vi "SLM_display A.vi"(1 "SLM Settings":T1={"resizeTo"=enum."Width of Display", "displayOn"=enum."All 3rd Monitor", "Top Left of Hologram"={"Horizontal"=60, "Vertical"=-210}}, 2 "SLM colour coding":enum16{"8-bit", "10-bit (Santec)"}(ring)=enum."10-bit (Santec)", 4 "Hologram":dbl[][](array[numeric])=array256x256[65536 elements]) -> (0 "SLM A":picture)   [LabVIEW 2024]
uses:
  typeDefs/slmSettings.ctl
  <vilib>/picture/picture.llb/Draw 8-Bit Pixmap.vi
  <vilib>/picture/picture.llb/Draw True-Color Pixmap.vi
panel:
  in  "Blazing Function 2":u8[](array[numeric])=[1, 2, 3, 4, 5, 6, 7, 8, 9, 10, 10, 11, 12, 13, 14, 15, 16, 17, 18, 19, 20, 21, 22, 23, 24, 25, 26, 27, 28, 29, 30, 31, 32, 32, 33, 34, 35, 36, 37, 38, 39, 40, 41, 42, 43, 44, 45, 46, 47, 48, 49, 50, 51, 52, 53, 54, 55, 56, 57, 58, 59, 60, 61, 61, 62, 63, 64, 65, 66, 67, 68, 69, 70, 71, 72, 73, 74, 75, 76, 77, 78, 79, 80, 81, 83, 84, 85, 86, 87, 88, 89, 90, 91, 92, 93, 94, 95, 96, 97, 98, 99, 100, 101, 102, 103, 104, 105, 106, 107, 108, 109, 111, 112, 113, 114, 115, 116, 117, 118, 119, 120, 121, 122, 123, 124, 125, 126, 127, 128, 129, 130, 131, 133, 134, 135, 136, 137, 138, 139, 140, 141, 142, 143, 144, 145, 146, 147, 148, 149, 150, 151, 152, 153, 154, 155, 156, 157, 158, 159, 160, 161, 162, 163, 164, 165, 166, 167, 168, 169, 170, 171, 172, 173, 174, 175, 176, 177, 178, 179, 180, 181, 182, 183, 184, 185, 186, 187, 188, 189, 190, 191, 192, 193, 194, 195, 196, 197, 198, 198, 199, 200, 201, 202, 203, 204, 205, 206, 207, 208, 209, 210, 211, 212, 213, 214, 215, 216, 217, 218, 219, 219, 220, 221, 222, 223, 224, 225, 226, 227, 228, 229, 230, 231, 232, 233, 234, 235, 236, 237, 238, 238, 239, 240, 241, 242, 243, 244, 245, 246, 247, 248, 249, 250, 251, 252, 253]
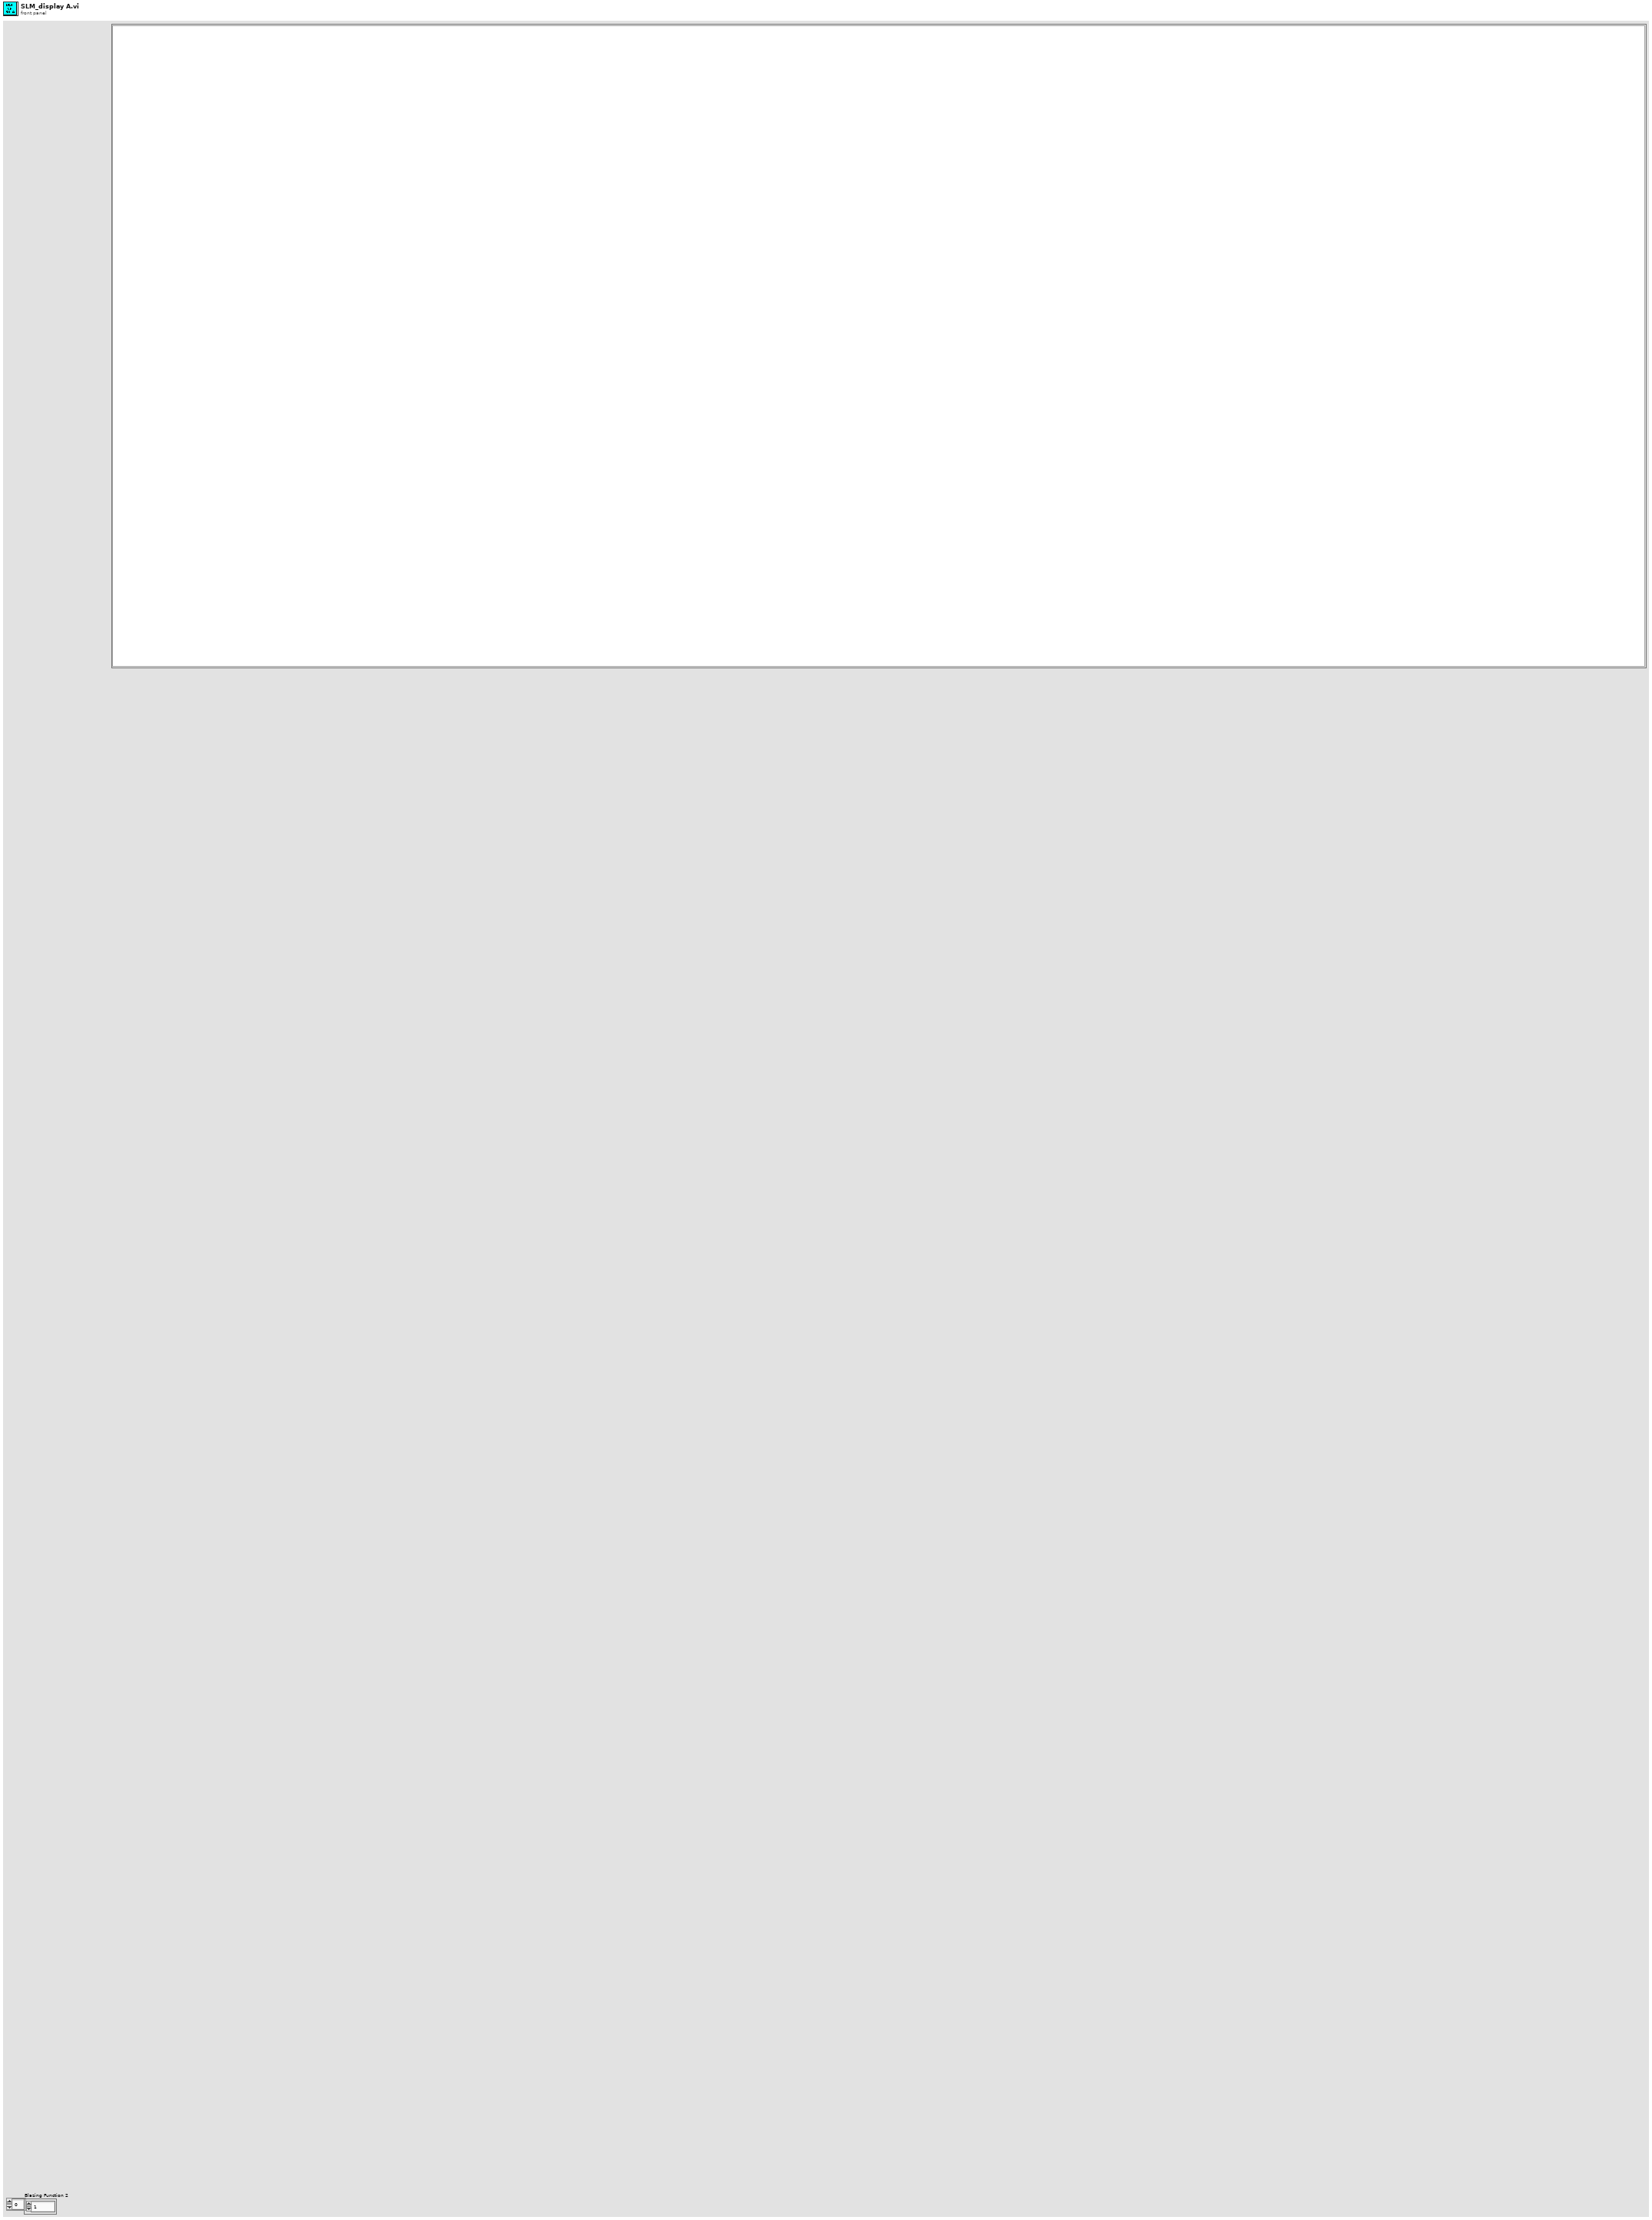
[diagram p1: front panel]
types:
  T1 = typedef "slmSettings.ctl" = cluster{"resizeTo":enum16{"No Resize", "Width of Display", "Height of Display"}, "displayOn":enum16{"Default", "All 1st Monitor", "All 2nd Monitor", "All 3rd Monitor", "All 4th Monitor"}, "Top Left of Hologram":cluster{"Horizontal":i16, "Vertical":i16}}
  T2 = enum16{"No Resize", "Width of Display", "Height of Display"}
  T3 = enum16{"Default", "All 1st Monitor", "All 2nd Monitor", "All 3rd Monitor", "All 4th Monitor"}
  T4 = typedef "LVRectTypeDef.ctl" = cluster{"Left":i16, "Top":i16, "Right":i16, "Bottom":i16}
  T5 = typedef "LVAllMonitorsDisplayTypeDef.ctl" = cluster{"Bounds":cluster{"Left":i16, "Top":i16, "Right":i16, "Bottom":i16}, "Depth":i16}[]
  T6 = cluster{"Bounds":cluster{"Left":i16, "Top":i16, "Right":i16, "Bottom":i16}, "Depth":i16}
  T7 = cluster{"Left":i16, "Top":i16, "Right":i16, "Bottom":i16}
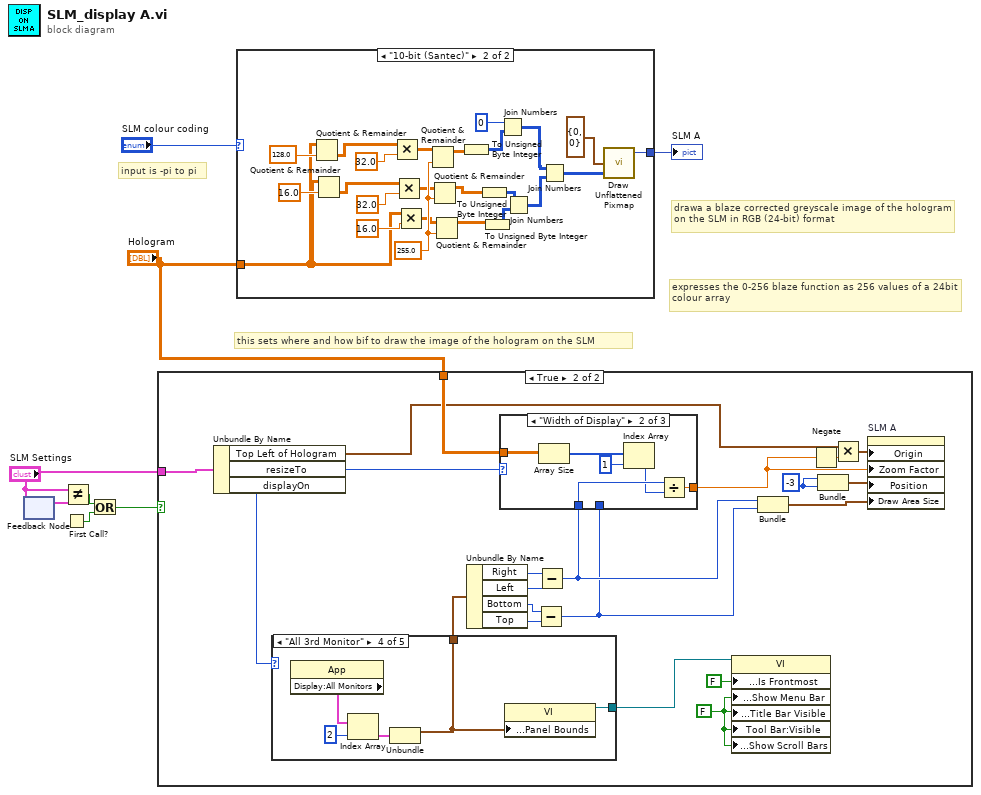
[diagram p0: block diagram]
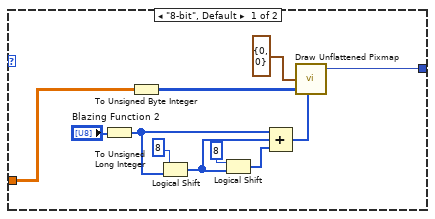
[diagram p2: hidden frame]
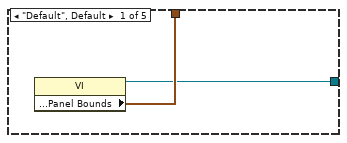
[diagram p4: hidden frame]
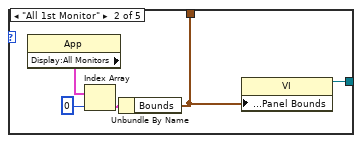
[diagram p5: hidden frame]
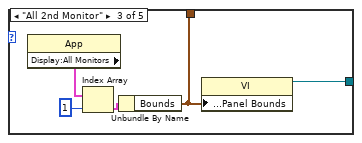
[diagram p6: hidden frame]
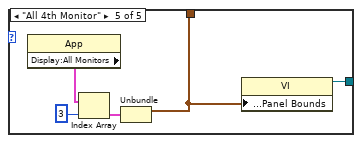
[diagram p7: hidden frame]
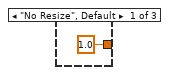
[diagram p8: hidden frame]
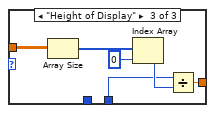
[diagram p9: hidden frame]
diagram:
  # "this sets where and how bif to draw the image of the hologram on the SLM"
  # "drawa a blaze corrected greyscale image of the hologram on the SLM in RGB (24-bit) format"
  # "input is -pi to pi"
  # "expresses the 0-256 blaze function as 256 values of a 24bit colour array"
  n1 = feedback-in #1("SLM Settings") -> ()
  n2 = feedback #1() -> (w8:T1)  [unwired: 1 in]
  n3 = First Call?() -> (First Call?: T/F=w7:bool)
  n4 = Not Equal?(x="SLM Settings", y=w8) -> (x != y?=w6:bool)
  n5 = Or(x=w6, y=w7) -> (x .or. y?=w5:bool)
  n6 = case shown="True" w5 {
    tunnel: "Hologram" -> [_ w24]
    tunnel: "SLM Settings" -> [_ w10]
    frame False {
    }
    frame True {
      w19 = i16 -3 ("x-y")
      w28 = FALSE ("Front Panel Window:Size To Screen")
      n7 = Unbundle By Name(w10) -> ("Top Left of Hologram"=w9:cluster{"Horizontal":i16, "Vertical":i16}, "resizeTo"=w26:T2, "displayOn"=w12:T3)
      n8 = case shown="\"All 3rd Monitor\"" w12 {
        tunnel: [w31 w33 w37 w43 w47] -> w27
        tunnel: [w30 w32 w38 w42 w48] -> w25
        frame "Default", Default {
          n9 = property class="VI"() -> (reference out=w30:refnum<vi>, "Front Panel Window:Panel Bounds"=w31:T4)  [unwired: 2 in, 1 out]
        }
        frame "All 1st Monitor" {
          n10 = property class="App"() -> ("Display:All Monitors"=w35:T5)  [unwired: 2 in, 2 out]
          n11 = Index Array(array=w35, index=0) -> (element=w34:T6)
          n12 = Unbundle By Name(w34) -> ("Bounds"=w33:T7)
          n13 = property class="VI"("Front Panel Window:Panel Bounds"=w33) -> (reference out=w32:refnum<vi>)  [unwired: 2 in, 1 out]
        }
        frame "All 2nd Monitor" {
          n14 = property class="App"() -> ("Display:All Monitors"=w40:T5)  [unwired: 2 in, 2 out]
          n15 = Index Array(array=w40, index=1) -> (element=w39:T6)
          n16 = Unbundle By Name(w39) -> ("Bounds"=w37:T7)
          n17 = property class="VI"("Front Panel Window:Panel Bounds"=w37) -> (reference out=w38:refnum<vi>)  [unwired: 2 in, 1 out]
        }
        frame "All 3rd Monitor" {
          n18 = property class="App"() -> ("Display:All Monitors"=w45:T5)  [unwired: 2 in, 2 out]
          n19 = Index Array(array=w45, index=2) -> (element=w44:T6)
          n20 = Unbundle(w44) -> ("Bounds"=w43:T7)  [unwired: 1 out]
          n21 = property class="VI"("Front Panel Window:Panel Bounds"=w43) -> (reference out=w42:refnum<vi>)  [unwired: 2 in, 1 out]
        }
        frame "All 4th Monitor" {
          n22 = property class="App"() -> ("Display:All Monitors"=w50:T5)  [unwired: 2 in, 2 out]
          n23 = Index Array(array=w50, index=3) -> (element=w49:T6)
          n24 = Unbundle(w49) -> ("Bounds"=w47:T7)  [unwired: 1 out]
          n25 = property class="VI"("Front Panel Window:Panel Bounds"=w47) -> (reference out=w48:refnum<vi>)  [unwired: 2 in, 1 out]
        }
      }
      n26 = Unbundle By Name(w27) -> ("Right"=w15:i16, "Left"=w14:i16, "Bottom"=w17:i16, "Top"=w16:i16)
      n27 = Subtract(x=w17, y=w16) -> (x-y=w11:i16)
      n28 = Subtract(x=w15, y=w14) -> (x-y=w13:i16)
      n29 = case shown="\"Width of Display\"" w26 {
        tunnel: w13 -> [_ w56 _]
        tunnel: [1.0 w55 w62] -> w23
        tunnel: w11 -> [_ _ w60]
        tunnel: w24 -> [_ w53 w59]
        frame "No Resize", Default {
        }
        frame "Width of Display" {
          n30 = Array Size(array=w53) -> (size(s)=w58:i32[])
          n31 = Index Array(array=w58, index=1) -> (element=w54:i32)
          n32 = Divide(x=w56, y=w54) -> (x/y=w55:dbl)
        }
        frame "Height of Display" {
          n33 = Array Size(array=w59) -> (size(s)=w64:i32[])
          n34 = Index Array(array=w64, index=0) -> (element=w61:i32)
          n35 = Divide(x=w60, y=w61) -> (x/y=w62:dbl)
        }
      }
      n36 = property class="VI"(reference=w25, "Front Panel Window:Is Frontmost"=FALSE ("Front Panel Window:Size To Screen"), "Front Panel Window:Show Menu Bar"=w28, "Front Panel Window:Title Bar Visible"=w28, "Tool Bar:Visible"=w28, "Front Panel Window:Show Scroll Bars"=w28) -> ()  [unwired: 1 in, 2 out]
      n37 = Bundle(w13, w11) -> (w20:cluster{i16, i16})  [unwired: 1 out]
      n38 = Negate(x=w23) -> (-x=w22:dbl)
      n39 = Bundle("x-y"=w19, "x-y"=w19) -> (w18:cluster{"x-y":i16, "x-y":i16})  [unwired: 1 out]
      n40 = Multiply(x=w9, y=w22) -> (x*y=w21:cluster{"Horizontal":dbl, "Vertical":dbl})
      n41 = property on="SLM A" class="Pict"("Origin"=w21, "Zoom Factor"=w23, "Position"=w18, "Draw Area Size"=w20) -> ()  [unwired: 2 in, 2 out]
    }
  }
  n42 = case shown="\"10-bit (Santec)\"" "SLM colour coding" {
    tunnel: [w67 w77] -> w4
    tunnel: "Hologram" -> [w66 w76]
    frame "8-bit", Default {
      n43 = To Unsigned Long Integer(number="Blazing Function 2") -> (unsigned 32bit integer=w65:u32[])
      n44 = To Unsigned Byte Integer(number=w66) -> (unsigned 8bit integer=w75:u8[][])
      n45 = Logical Shift(y=8, x=w65) -> (x << y=w73:u32[])
      n46 = Logical Shift(y=8, x=w73) -> (x << y=w72:u32[])
      n47 = Compound Arithmetic op=ADD(w65, w73, w72) -> (w74:u32[])
      n48 = call-poly <vilib>:"Draw Unflattened Pixmap.vi"("top left point(0, 0)"=cluster{"x":i16, "y":i16} {"x"=0, "y"=0}, "data"=w75, "color table"=w74) -> ("new picture"=w67:picture)  [unwired: 2 in, 4 out]
    }
    frame "10-bit (Santec)" {
      w85 = 255.0
      n49 = Quotient & Remainder(x=w76, y=128.0) -> (floor(x/y)=w97:dbl[][])  [unwired: 1 out]
      n50 = Quotient & Remainder(x=w76, y=16.0) -> (floor(x/y)=w95:dbl[][])  [unwired: 1 out]
      n51 = Multiply(x=w97, y=32.0) -> (x*y=w84:dbl[][])
      n52 = Multiply(x=w95, y=32.0) -> (x*y=w83:dbl[][])
      n53 = Multiply(x=w76, y=16.0) -> (x*y=w82:dbl[][])
      n54 = Quotient & Remainder(x=w84, y=w85) -> (x-y*floor(x/y)=w81:dbl[][])  [unwired: 1 out]
      n55 = Quotient & Remainder(x=w83, y=w85) -> (x-y*floor(x/y)=w80:dbl[][])  [unwired: 1 out]
      n56 = Quotient & Remainder(x=w82, y=w85) -> (x-y*floor(x/y)=w79:dbl[][])  [unwired: 1 out]
      n57 = To Unsigned Byte Integer(number=w81) -> (unsigned 8bit integer=w88:u8[][])
      n58 = To Unsigned Byte Integer(number=w80) -> (unsigned 8bit integer=w87:u8[][])
      n59 = To Unsigned Byte Integer(number=w79) -> (unsigned 8bit integer=w86:u8[][])
      n60 = Join Numbers(hi=u8 0, lo=w88) -> ((hi.lo)=w91:u16[][])
      n61 = Join Numbers(hi=w87, lo=w86) -> ((hi.lo)=w90:u16[][])
      n62 = Join Numbers(hi=w91, lo=w90) -> ((hi.lo)=w89:u32[][])
      n63 = call-poly <vilib>:"Draw Unflattened Pixmap.vi"("top left point(0, 0)"=cluster{"x":i16, "y":i16} {"x"=0, "y"=0}, "data (RGB format)"=w89) -> ("new picture"=w77:picture)  [unwired: 2 in, 5 out]
    }
  }
  "SLM A" <- w4
